vi "UTF8 to ANS_DKI.vi"(3 "error in":errorcluster, 4 "Code Page":i32(ring) items=["System default"=0, "Latin-1"=1252, "Japanese"=932, "Korean"=947, "Chinese simplified"=936, "Chinese traditional"=950, "Central Europe"=1250, "Cyrillic"=1251, "Greek"=1253, "Turkish"=1254, "Hebrew"=1255, "Arabic"=1256, "Baltic"=1257, "Thai"=874, "Vietnamese"=783, "UTF8"=65001, "UTF-7"=65000], 5 "UTF8 string":string="tété") -> (0 "error out":errorcluster, 2 "ANSI/Multibyte string":string="tété")   [LabVIEW 2024]
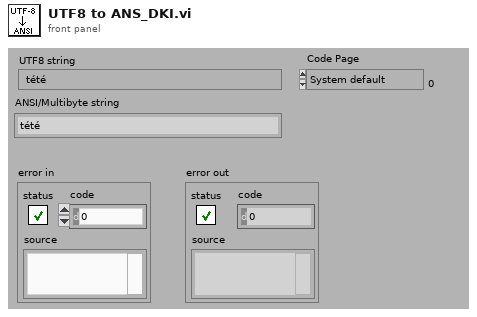
[diagram p1: front panel]
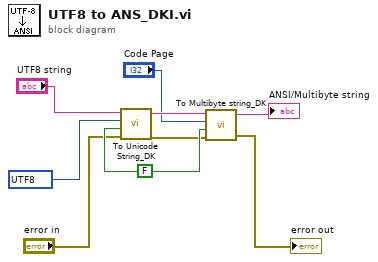
[diagram p0: block diagram]
diagram:
  w8 = FALSE ("Big Endian?")
  w6 = 65001 items=["System default"=0, "Latin-1"=1252, "Japanese"=932, "Korean"=947, "Chinese simplified"=936, "Chinese traditional"=950, "Central Europe"=1250, "Cyrillic"=1251, "Greek"=1253, "Turkish"=1254, "Hebrew"=1255, "Arabic"=1256, "Baltic"=1257, "Thai"=874, "Vietnamese"=783, "UTF8"=65001, "UTF-7"=65000] ("Code Page")
  n1 = call "To Unicode String_DK.vi"("error in"="error in", "Big Endian?"=w8, "Code Page"=w6, "Multibyte String"="UTF8 string") -> ("error out"=w1:errorcluster, "Unicode string"=w4:string)  [unwired: 1 out]
  n2 = call "To Multibyte string_DK.vi"("error in"=w1, "Big Endian?"=w8, "Code Page"="Code Page", "Unicode String"=w4) -> ("error out"=→"error out":errorcluster, "Multibyte string"=→"ANSI/Multibyte string":string)  [unwired: 1 out]
